vi "Write DAQ FIFO.vi"(6 "FIFO Timestamps":T2, 8 "error in (no error)":errorcluster, 9 "Timeout (ms)":i32=100, 10 "Data In":T1[](array[typedef]), 11 "CIF_DAQ_DVR_Multi in":refnum<class "CIF_DAQ_DVR_Multi.lvclass">) -> (0 "error out":errorcluster, 1 "timed out?":bool, 2 "Data Out":T1[](array[typedef]), 3 "CIF_DAQ_DVR_Multi out":refnum<class "CIF_DAQ_DVR_Multi.lvclass">)   [LabVIEW 2021, in "CIF_DAQ_DVR_Multi.lvclass"]
uses:
  CIF_DAQ_DVR_Multi.lvclass
  ChannelCommon/typedef/TimeStamps.ctl
  ChannelCommon/typedef/Datatype Waveform.ctl
  CIF_DAQ_DVR_Multi.lvclass/CIF_DAQ_DVR_Multi.ctl
  FIFO_DAQ_DVR/CIF_NIChn_FIFO_DAQ_DVR.lvclass
  CIFChannels/CIFChannels.lvclass
  369b2d9f-cd2a-4ce2-92c3-19653a73c8ad.vi
  e6281684-375c-44a7-85bc-c0cc59c3c0f1.vi
  D:/dev/Packages/Channel_Manager/src/CIF_NIChn/FIFO_DAQ_DVR/CIF_NIChn_FIFO_DAQ_DVR.lvclass
  D:/dev/Packages/Channel_Manager/src/CIF_NIChn/FIFO_U8/CIF_NIChn_Fifo_U8.lvclass
  D:/dev/Packages/Channel_Manager/src/CIF_NIChn/NIChn/CIF_NIChn.lvclass
  D:/dev/Packages/Channel_Manager/src/CIFChannels/CIFChannels.lvclass
  D:/dev/Packages/Channel_Manager/src/CIF_NIChn/FIFO_DAQ_DVR_Multi/CIF_DAQ_DVR_Multi.lvclass
  ChannelCommon/ChannelCommon.lvlib
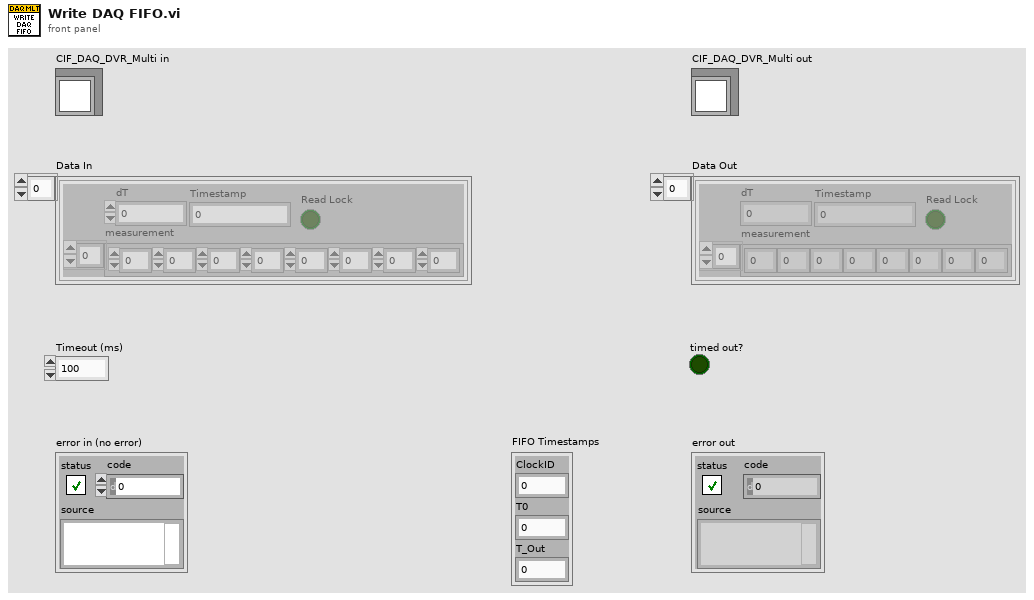
[diagram p1: front panel]
types:
  T1 = typedef "ChannelCommon.lvlib/Datatype Waveform.ctl" = cluster{"measurement":dbl[], "dT":dbl, "Timestamp":i64, "Read Lock":bool}
  T2 = typedef "ChannelCommon.lvlib/TimeStamps.ctl" = cluster{"ClockID":u8, "T0":i64, "T_Out":i64}
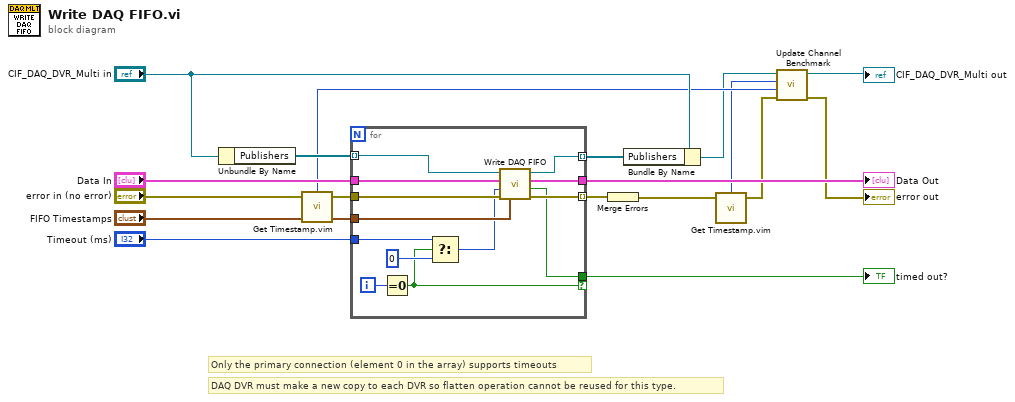
[diagram p0: block diagram]
diagram:
  # "Only the primary connection (element 0 in the array) supports timeouts"
  # "DAQ DVR must make a new copy to each DVR so flatten operation cannot be reused for this type."
  n1 = Unbundle By Name("CIF_DAQ_DVR_Multi in") -> ("Publishers"=w18:refnum<class "CIF_NIChn_FIFO_DAQ_DVR.lvclass">[])
  n2 = call "Get Timestamp.vim"("Anything in"="error in (no error)") -> ("Time (ns)"=w9:i64, "Anything out"=w5:errorcluster)  [unwired: 2 in]
  n3 = for {
    tunnel: w18 -> [w31] mode=indexing
    tunnel: "Data In" -> [w30]
    tunnel: [w29] -> w16
    tunnel: [w28] -> w14 mode=indexing
    tunnel: [w27] -> w13 mode=indexing
    tunnel: w5 -> [w26]
    tunnel: "FIFO Timestamps" -> [w25]
    tunnel: "Timeout (ms)" -> [w23]
    tunnel: [w20] -> w10 if=w19
    i -> [w24]
    n4 = Equal To 0?(x=w24) -> (x = 0?=w19:bool)
    n5 = Select(t=w23, s=w19, f=0) -> (s? t:f=w22:i32)
    n6 = call-dynamic "Write DAQ FIFO.vi"("FIFO Timestamps"=w25, "error in (no error)"=w26, "Timeout (ms)"=w22, "Data In"=w30, "CIF_NIChn_FIFO_DAQ in"=w31) -> ("error out"=w27:errorcluster, "timed out?"=w20:bool, "Data Out"=w29:T1[], "CIF_NIChn_FIFO_DAQ out"=w28:refnum<class "CIF_NIChn_FIFO_DAQ_DVR.lvclass">)  [unwired: 3 in]
  }
  "timed out?" <- w10
  "Data Out" <- w16
  n7 = Merge Errors(w13) -> (w4:errorcluster)
  n8 = Bundle By Name(cluster="CIF_DAQ_DVR_Multi in", "Publishers"=w14) -> (w2:refnum<class "CIF_DAQ_DVR_Multi.lvclass">)
  n9 = call "Get Timestamp.vim"("Anything in"=w4) -> ("Time (ns)"=w8:i64, "Anything out"=w7:errorcluster)  [unwired: 2 in]
  n10 = call "Update Channel Benchmark.vi"("error in (no error)"=w7, "X0"=w9, "X1"=w8, "CIFChannels in"=w2) -> ("error out"=→"error out":errorcluster, "CIFChannels out"=→"CIF_DAQ_DVR_Multi out":refnum<class "CIF_DAQ_DVR_Multi.lvclass">)  [unwired: 6 in]
